vi "logical operations.vi"() -> ()   [LabVIEW 2017]
panel:
  out "EXOR":bool
  out "OR":bool
  out "AND":bool
  in  "B":bool
  in  "A":bool
  # "1"
  # "1"
  # "1"
  # "1"
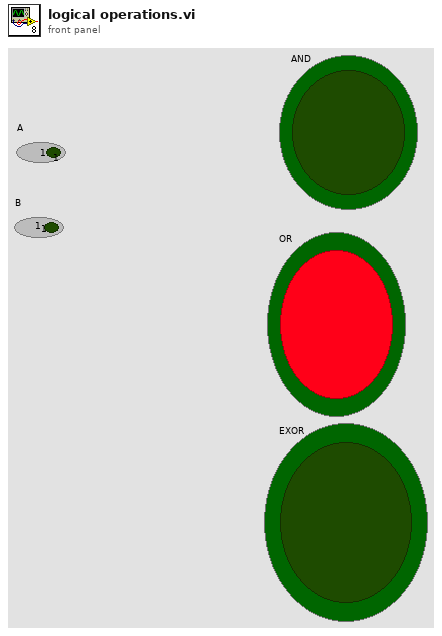
[diagram p1: front panel]
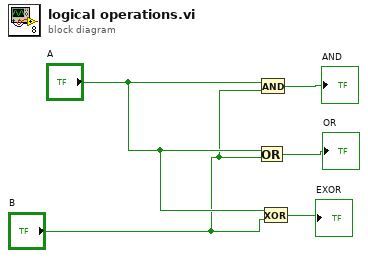
[diagram p0: block diagram]
diagram:
  n1 = Or(x="A", y="B") -> (x .or. y?=→"OR":bool)
  n2 = And(x="A", y="B") -> (x .and. y?=→"AND":bool)
  n3 = Exclusive Or(1:"B", 2:"A") -> (0:→"EXOR":bool)
